vi "FipsAdjacent.vi"() -> (11 "Fips":i32[](array[numeric]))   [LabVIEW 2017] (continued)
 SD\"\t46127\t\"Sioux County, IA\"\t19167\n\"Union County, SD\"\t46127\t\"Woodbury County, IA\"\t19193\n\"Union County, SD\"\t46127\t\"Dakota County, NE\"\t31043\n\"Union County, SD\"\t46127\t\"Dixon County, NE\"\t31051\n\"Union County, SD\"\t46127\t\"Clay County, SD\"\t46027\n\"Union County, SD\"\t46127\t\"Lincoln County, SD\"\t46083\n\"Union County, SD\"\t46127\t\"Union County, SD\"\t46127\n\"Walworth County, SD\"\t46129\t\"Campbell County, SD\"\t46021\n\"Walworth County, SD\"\t46129\t\"Corson County, SD\"\t46031\n\"Walworth County, SD\"\t46129\t\"Dewey County, SD\"\t46041\n\"Walworth County, SD\"\t46129\t\"Edmunds County, SD\"\t46045\n\"Walworth County, SD\"\t46129\t\"McPherson County, SD\"\t46089\n\"Walworth County, SD\"\t46129\t\"Potter County, SD\"\t46107\n\"Walworth County, SD\"\t46129\t\"Walworth County, SD\"\t46129\n\"Yankton County, SD\"\t46135\t\"Cedar County, NE\"\t31027\n\"Yankton County, SD\"\t46135\t\"Knox County, NE\"\t31107\n\"Yankton County, SD\"\t46135\t\"Bon Homme County, SD\"\t46009\n\"Yankton County, SD\"\t46135\t\"Clay County, SD\"\t46027\n\"Yankton County, SD\"\t46135\t\"Hutchinson County, SD\"\t46067\n\"Yankton County, SD\"\t46135\t\"Turner County, SD\"\t46125\n\"Yankton County, SD\"\t46135\t\"Yankton County, SD\"\t46135\n\"Ziebach County, SD\"\t46137\t\"Corson County, SD\"\t46031\n\"Ziebach County, SD\"\t46137\t\"Dewey County, SD\"\t46041\n\"Ziebach County, SD\"\t46137\t\"Haakon County, SD\"\t46055\n\"Ziebach County, SD\"\t46137\t\"Meade County, SD\"\t46093\n\"Ziebach County, SD\"\t46137\t\"Perkins County, SD\"\t46105\n\"Ziebach County, SD\"\t46137\t\"Stanley County, SD\"\t46117\n\"Ziebach County, SD\"\t46137\t\"Ziebach County, SD\"\t46137\n\"Anderson County, TN\"\t47001\t\"Anderson County, TN\"\t47001\n\"Anderson County, TN\"\t47001\t\"Campbell County, TN\"\t47013\n\"Anderson County, TN\"\t47001\t\"Knox County, TN\"\t47093\n\"Anderson County, TN\"\t47001\t\"Morgan County, TN\"\t47129\n\"Anderson County, TN\"\t47001\t\"Roane County, TN\"\t47145\n\"Anderson County, TN\"\t47001\t\"Scott County, TN\"\t47151\n\"Anderson County, TN\"\t47001\t\"Union County, TN\"\t47173\n\"Bedford County, TN\"\t47003\t\"Bedford County, TN\"\t47003\n\"Bedford County, TN\"\t47003\t\"Coffee County, TN\"\t47031\n\"Bedford County, TN\"\t47003\t\"Lincoln County, TN\"\t47103\n\"Bedford County, TN\"\t47003\t\"Marshall County, TN\"\t47117\n\"Bedford County, TN\"\t47003\t\"Moore County, TN\"\t47127\n\"Bedford County, TN\"\t47003\t\"Rutherford County, TN\"\t47149\n\"Benton County, TN\"\t47005\t\"Benton County, TN\"\t47005\n\"Benton County, TN\"\t47005\t\"Carroll County, TN\"\t47017\n\"Benton County, TN\"\t47005\t\"Decatur County, TN\"\t47039\n\"Benton County, TN\"\t47005\t\"Henry County, TN\"\t47079\n\"Benton County, TN\"\t47005\t\"Houston County, TN\"\t47083\n\"Benton County, TN\"\t47005\t\"Humphreys County, TN\"\t47085\n\"Benton County, TN\"\t47005\t\"Perry County, TN\"\t47135\n\"Benton County, TN\"\t47005\t\"Stewart County, TN\"\t47161\n\"Bledsoe County, TN\"\t47007\t\"Bledsoe County, TN\"\t47007\n\"Bledsoe County, TN\"\t47007\t\"Cumberland County, TN\"\t47035\n\"Bledsoe County, TN\"\t47007\t\"Hamilton County, TN\"\t47065\n\"Bledsoe County, TN\"\t47007\t\"Rhea County, TN\"\t47143\n\"Bledsoe County, TN\"\t47007\t\"Sequatchie County, TN\"\t47153\n\"Bledsoe County, TN\"\t47007\t\"Van Buren County, TN\"\t47175\n\"Blount County, TN\"\t47009\t\"Graham County, NC\"\t37075\n\"Blount County, TN\"\t47009\t\"Swain County, NC\"\t37173\n\"Blount County, TN\"\t47009\t\"Blount County, TN\"\t47009\n\"Blount County, TN\"\t47009\t\"Knox County, TN\"\t47093\n\"Blount County, TN\"\t47009\t\"Loudon County, TN\"\t47105\n\"Blount County, TN\"\t47009\t\"Monroe County, TN\"\t47123\n\"Blount County, TN\"\t47009\t\"Sevier County, TN\"\t47155\n\"Bradley County, TN\"\t47011\t\"Murray County, GA\"\t13213\n\"Bradley County, TN\"\t47011\t\"Whitfield County, GA\"\t13313\n\"Bradley County, TN\"\t47011\t\"Bradley County, TN\"\t47011\n\"Bradley County, TN\"\t47011\t\"Hamilton County, TN\"\t47065\n\"Bradley County, TN\"\t47011\t\"McMinn County, TN\"\t47107\n\"Bradley County, TN\"\t47011\t\"Meigs County, TN\"\t47121\n\"Bradley County, TN\"\t47011\t\"Polk County, TN\"\t47139\n\"Campbell County, TN\"\t47013\t\"McCreary County, KY\"\t21147\n\"Campbell County, TN\"\t47013\t\"Whitley County, KY\"\t21235\n\"Campbell County, TN\"\t47013\t\"Anderson County, TN\"\t47001\n\"Campbell County, TN\"\t47013\t\"Campbell County, TN\"\t47013\n\"Campbell County, TN\"\t47013\t\"Claiborne County, TN\"\t47025\n\"Campbell County, TN\"\t47013\t\"Scott County, TN\"\t47151\n\"Campbell County, TN\"\t47013\t\"Union County, TN\"\t47173\n\"Cannon County, TN\"\t47015\t\"Cannon County, TN\"\t47015\n\"Cannon County, TN\"\t47015\t\"Coffee County, TN\"\t47031\n\"Cannon County, TN\"\t47015\t\"DeKalb County, TN\"\t47041\n\"Cannon County, TN\"\t47015\t\"Rutherford County, TN\"\t47149\n\"Cannon County, TN\"\t47015\t\"Warren County, TN\"\t47177\n\"Cannon County, TN\"\t47015\t\"Wilson County, TN\"\t47189\n\"Carroll County, TN\"\t47017\t\"Benton County, TN\"\t47005\n\"Carroll County, TN\"\t47017\t\"Carroll County, TN\"\t47017\n\"Carroll County, TN\"\t47017\t\"Decatur County, TN\"\t47039\n\"Carroll County, TN\"\t47017\t\"Gibson County, TN\"\t47053\n\"Carroll County, TN\"\t47017\t\"Henderson County, TN\"\t47077\n\"Carroll County, TN\"\t47017\t\"Henry County, TN\"\t47079\n\"Carroll County, TN\"\t47017\t\"Madison County, TN\"\t47113\n\"Carroll County, TN\"\t47017\t\"Weakley County, TN\"\t47183\n\"Carter County, TN\"\t47019\t\"Avery County, NC\"\t37011\n\"Carter County, TN\"\t47019\t\"Mitchell County, NC\"\t37121\n\"Carter County, TN\"\t47019\t\"Carter County, TN\"\t47019\n\"Carter County, TN\"\t47019\t\"Johnson County, TN\"\t47091\n\"Carter County, TN\"\t47019\t\"Sullivan County, TN\"\t47163\n\"Carter County, TN\"\t47019\t\"Unicoi County, TN\"\t47171\n\"Carter County, TN\"\t47019\t\"Washington County, TN\"\t47179\n\"Cheatham County, TN\"\t47021\t\"Cheatham County, TN\"\t47021\n\"Cheatham County, TN\"\t47021\t\"Davidson County, TN\"\t47037\n\"Cheatham County, TN\"\t47021\t\"Dickson County, TN\"\t47043\n\"Cheatham County, TN\"\t47021\t\"Montgomery County, TN\"\t47125\n\"Cheatham County, TN\"\t47021\t\"Robertson County, TN\"\t47147\n\"Cheatham County, TN\"\t47021\t\"Williamson County, TN\"\t47187\n\"Chester County, TN\"\t47023\t\"Chester County, TN\"\t47023\n\"Chester County, TN\"\t47023\t\"Hardeman County, TN\"\t47069\n\"Chester County, TN\"\t47023\t\"Hardin County, TN\"\t47071\n\"Chester County, TN\"\t47023\t\"Henderson County, TN\"\t47077\n\"Chester County, TN\"\t47023\t\"McNairy County, TN\"\t47109\n\"Chester County, TN\"\t47023\t\"Madison County, TN\"\t47113\n\"Claiborne County, TN\"\t47025\t\"Bell County, KY\"\t21013\n\"Claiborne County, TN\"\t47025\t\"Whitley County, KY\"\t21235\n\"Claiborne County, TN\"\t47025\t\"Campbell County, TN\"\t47013\n\"Claiborne County, TN\"\t47025\t\"Claiborne County, TN\"\t47025\n\"Claiborne County, TN\"\t47025\t\"Grainger County, TN\"\t47057\n\"Claiborne County, TN\"\t47025\t\"Hancock County, TN\"\t47067\n\"Claiborne County, TN\"\t47025\t\"Union County, TN\"\t47173\n\"Claiborne County, TN\"\t47025\t\"Lee County, VA\"\t51105\n\"Clay County, TN\"\t47027\t\"Clinton County, KY\"\t21053\n\"Clay County, TN\"\t47027\t\"Cumberland County, KY\"\t21057\n\"Clay County, TN\"\t47027\t\"Monroe County, KY\"\t21171\n\"Clay County, TN\"\t47027\t\"Clay County, TN\"\t47027\n\"Clay County, TN\"\t47027\t\"Jackson County, TN\"\t47087\n\"Clay County, TN\"\t47027\t\"Macon County, TN\"\t47111\n\"Clay County, TN\"\t47027\t\"Overton County, TN\"\t47133\n\"Clay County, TN\"\t47027\t\"Pickett County, TN\"\t47137\n\"Cocke County, TN\"\t47029\t\"Haywood County, NC\"\t37087\n\"Cocke County, TN\"\t47029\t\"Madison County, NC\"\t37115\n\"Cocke County, TN\"\t47029\t\"Cocke County, TN\"\t47029\n\"Cocke County, TN\"\t47029\t\"Greene County, TN\"\t47059\n\"Cocke County, TN\"\t47029\t\"Hamblen County, TN\"\t47063\n\"Cocke County, TN\"\t47029\t\"Jefferson County, TN\"\t47089\n\"Cocke County, TN\"\t47029\t\"Sevier County, TN\"\t47155\n\"Coffee County, TN\"\t47031\t\"Bedford County, TN\"\t47003\n\"Coffee County, TN\"\t47031\t\"Cannon County, TN\"\t47015\n\"Coffee County, TN\"\t47031\t\"Coffee County, TN\"\t47031\n\"Coffee County, TN\"\t47031\t\"Franklin County, TN\"\t47051\n\"Coffee County, TN\"\t47031\t\"Grundy County, TN\"\t47061\n\"Coffee County, TN\"\t47031\t\"Moore County, TN\"\t47127\n\"Coffee County, TN\"\t47031\t\"Rutherford County, TN\"\t47149\n\"Coffee County, TN\"\t47031\t\"Warren County, TN\"\t47177\n\"Crockett County, TN\"\t47033\t\"Crockett County, TN\"\t47033\n\"Crockett County, TN\"\t47033\t\"Dyer County, TN\"\t47045\n\"Crockett County, TN\"\t47033\t\"Gibson County, TN\"\t47053\n\"Crockett County, TN\"\t47033\t\"Haywood County, TN\"\t47075\n\"Crockett County, TN\"\t47033\t\"Lauderdale County, TN\"\t47097\n\"Crockett County, TN\"\t47033\t\"Madison County, TN\"\t47113\n\"Cumberland County, TN\"\t47035\t\"Bledsoe County, TN\"\t47007\n\"Cumberland County, TN\"\t47035\t\"Cumberland County, TN\"\t47035\n\"Cumberland County, TN\"\t47035\t\"Fentress County, TN\"\t47049\n\"Cumberland County, TN\"\t47035\t\"Morgan County, TN\"\t47129\n\"Cumberland County, TN\"\t47035\t\"Putnam County, TN\"\t47141\n\"Cumberland County, TN\"\t47035\t\"Rhea County, TN\"\t47143\n\"Cumberland County, TN\"\t47035\t\"Roane County, TN\"\t47145\n\"Cumberland County, TN\"\t47035\t\"Van Buren County, TN\"\t47175\n\"Cumberland County, TN\"\t47035\t\"White County, TN\"\t47185\n\"Davidson County, TN\"\t47037\t\"Cheatham County, TN\"\t47021\n\"Davidson County, TN\"\t47037\t\"Davidson County, TN\"\t47037\n\"Davidson County, TN\"\t47037\t\"Robertson County, TN\"\t47147\n\"Davidson County, TN\"\t47037\t\"Rutherford County, TN\"\t47149\n\"Davidson County, TN\"\t47037\t\"Sumner County, TN\"\t47165\n\"Davidson County, TN\"\t47037\t\"Williamson County, TN\"\t47187\n\"Davidson County, TN\"\t47037\t\"Wilson County, TN\"\t47189\n\"Decatur County, TN\"\t47039\t\"Benton County, TN\"\t47005\n\"Decatur County, TN\"\t47039\t\"Carroll County, TN\"\t47017\n\"Decatur County, TN\"\t47039\t\"Decatur County, TN\"\t47039\n\"Decatur County, TN\"\t47039\t\"Hardin County, TN\"\t47071\n\"Decatur County, TN\"\t47039\t\"Henderson County, TN\"\t47077\n\"Decatur County, TN\"\t47039\t\"Perry County, TN\"\t47135\n\"Decatur County, TN\"\t47039\t\"Wayne County, TN\"\t47181\n\"DeKalb County, TN\"\t47041\t\"Cannon County, TN\"\t47015\n\"DeKalb County, TN\"\t47041\t\"DeKalb County, TN\"\t47041\n\"DeKalb County, TN\"\t47041\t\"Putnam County, TN\"\t47141\n\"DeKalb County, TN\"\t47041\t\"Smith County, TN\"\t47159\n\"DeKalb County, TN\"\t47041\t\"Warren County, TN\"\t47177\n\"DeKalb County, TN\"\t47041\t\"White County, TN\"\t47185\n\"DeKalb County, TN\"\t47041\t\"Wilson County, TN\"\t47189\n\"Dickson County, TN\"\t47043\t\"Cheatham County, TN\"\t47021\n\"Dickson County, TN\"\t47043\t\"Dickson County, TN\"\t47043\n\"Dickson County, TN\"\t47043\t\"Hickman County, TN\"\t47081\n\"Dickson County, TN\"\t47043\t\"Houston County, TN\"\t47083\n\"Dickson County, TN\"\t47043\t\"Humphreys County, TN\"\t47085\n\"Dickson County, TN\"\t47043\t\"Montgomery County, TN\"\t47125\n\"Dickson County, TN\"\t47043\t\"Williamson County, TN\"\t47187\n\"Dyer County, TN\"\t47045\t\"Mississippi County, AR\"\t05093\n\"Dyer County, TN\"\t47045\t\"Pemiscot County, MO\"\t29155\n\"Dyer County, TN\"\t47045\t\"Crockett County, TN\"\t47033\n\"Dyer County, TN\"\t47045\t\"Dyer County, TN\"\t47045\n\"Dyer County, TN\"\t47045\t\"Gibson County, TN\"\t47053\n\"Dyer County, TN\"\t47045\t\"Lake County, TN\"\t47095\n\"Dyer County, TN\"\t47045\t\"Lauderdale County, TN\"\t47097\n\"Dyer County, TN\"\t47045\t\"Obion County, TN\"\t47131\n\"Fayette County, TN\"\t47047\t\"Benton County, MS\"\t28009\n\"Fayette County, TN\"\t47047\t\"Marshall County, MS\"\t28093\n\"Fayette County, TN\"\t47047\t\"Fayette County, TN\"\t47047\n\"Fayette County, TN\"\t47047\t\"Hardeman County, TN\"\t47069\n\"Fayette County, TN\"\t47047\t\"Haywood County, TN\"\t47075\n\"Fayette County, TN\"\t47047\t\"Shelby County, TN\"\t47157\n\"Fayette County, TN\"\t47047\t\"Tipton County, TN\"\t47167\n\"Fentress County, TN\"\t47049\t\"Cumberland County, TN\"\t47035\n\"Fentress County, TN\"\t47049\t\"Fentress County, TN\"\t47049\n\"Fentress County, TN\"\t47049\t\"Morgan County, TN\"\t47129\n\"Fentress County, TN\"\t47049\t\"Overton County, TN\"\t47133\n\"Fentress County, TN\"\t47049\t\"Pickett County, TN\"\t47137\n\"Fentress County, TN\"\t47049\t\"Putnam County, TN\"\t47141\n\"Fentress County, TN\"\t47049\t\"Scott County, TN\"\t47151\n\"Franklin County, TN\"\t47051\t\"Jackson County, AL\"\t01071\n\"Franklin County, TN\"\t47051\t\"Madison County, AL\"\t01089\n\"Franklin County, TN\"\t47051\t\"Coffee County, TN\"\t47031\n\"Franklin County, TN\"\t47051\t\"Franklin County, TN\"\t47051\n\"Franklin County, TN\"\t47051\t\"Grundy County, TN\"\t47061\n\"Franklin County, TN\"\t47051\t\"Lincoln County, TN\"\t47103\n\"Franklin County, TN\"\t47051\t\"Marion County, TN\"\t47115\n\"Franklin County, TN\"\t47051\t\"Moore County, TN\"\t47127\n\"Gibson County, TN\"\t47053\t\"Carroll County, TN\"\t47017\n\"Gibson County, TN\"\t47053\t\"Crockett County, TN\"\t47033\n\"Gibson County, TN\"\t47053\t\"Dyer County, TN\"\t47045\n\"Gibson County, TN\"\t47053\t\"Gibson County, TN\"\t47053\n\"Gibson County, TN\"\t47053\t\"Madison County, TN\"\t47113\n\"Gibson County, TN\"\t47053\t\"Obion County, TN\"\t47131\n\"Gibson County, TN\"\t47053\t\"Weakley County, TN\"\t47183\n\"Giles County, TN\"\t47055\t\"Lauderdale County, AL\"\t01077\n\"Giles County, TN\"\t47055\t\"Limestone County, AL\"\t01083\n\"Giles County, TN\"\t47055\t\"Giles County, TN\"\t47055\n\"Giles County, TN\"\t47055\t\"Lawrence County, TN\"\t47099\n\"Giles County, TN\"\t47055\t\"Lincoln County, TN\"\t47103\n\"Giles County, TN\"\t47055\t\"Marshall County, TN\"\t47117\n\"Giles County, TN\"\t47055\t\"Maury County, TN\"\t47119\n\"Grainger County, TN\"\t47057\t\"Claiborne County, TN\"\t47025\n\"Grainger County, TN\"\t47057\t\"Grainger County, TN\"\t47057\n\"Grainger County, TN\"\t47057\t\"Hamblen County, TN\"\t47063\n\"Grainger County, TN\"\t47057\t\"Hancock County, TN\"\t47067\n\"Grainger County, TN\"\t47057\t\"Hawkins County, TN\"\t47073\n\"Grainger County, TN\"\t47057\t\"Jefferson County, TN\"\t47089\n\"Grainger County, TN\"\t47057\t\"Knox County, TN\"\t47093\n\"Grainger County, TN\"\t47057\t\"Union County, TN\"\t47173\n\"Greene County, TN\"\t47059\t\"Madison County, NC\"\t37115\n\"Greene County, TN\"\t47059\t\"Cocke County, TN\"\t47029\n\"Greene County, TN\"\t47059\t\"Greene County, TN\"\t47059\n\"Greene County, TN\"\t47059\t\"Hamblen County, TN\"\t47063\n\"Greene County, TN\"\t47059\t\"Hawkins County, TN\"\t47073\n\"Greene County, TN\"\t47059\t\"Unicoi County, TN\"\t47171\n\"Greene County, TN\"\t47059\t\"Washington County, TN\"\t47179\n\"Grundy County, TN\"\t47061\t\"Coffee County, TN\"\t47031\n\"Grundy County, TN\"\t47061\t\"Franklin County, TN\"\t47051\n\"Grundy County, TN\"\t47061\t\"Grundy County, TN\"\t47061\n\"Grundy County, TN\"\t47061\t\"Marion County, TN\"\t47115\n\"Grundy County, TN\"\t47061\t\"Sequatchie County, TN\"\t47153\n\"Grundy County, TN\"\t47061\t\"Warren County, TN\"\t47177\n\"Hamblen County, TN\"\t47063\t\"Cocke County, TN\"\t47029\n\"Hamblen County, TN\"\t47063\t\"Grainger County, TN\"\t47057\n\"Hamblen County, TN\"\t47063\t\"Greene County, TN\"\t47059\n\"Hamblen County, TN\"\t47063\t\"Hamblen County, TN\"\t47063\n\"Hamblen County, TN\"\t47063\t\"Hawkins County, TN\"\t47073\n\"Hamblen County, TN\"\t47063\t\"Jefferson County, TN\"\t47089\n\"Hamilton County, TN\"\t47065\t\"Catoosa County, GA\"\t13047\n\"Hamilton County, TN\"\t47065\t\"Dade County, GA\"\t13083\n\"Hamilton County, TN\"\t47065\t\"Walker County, GA\"\t13295\n\"Hamilton County, TN\"\t47065\t\"Whitfield County, GA\"\t13313\n\"Hamilton County, TN\"\t47065\t\"Bledsoe County, TN\"\t47007\n\"Hamilton County, TN\"\t47065\t\"Bradley County, TN\"\t47011\n\"Hamilton County, TN\"\t47065\t\"Hamilton County, TN\"\t47065\n\"Hamilton County, TN\"\t47065\t\"Marion County, TN\"\t47115\n\"Hamilton County, TN\"\t47065\t\"Meigs County, TN\"\t47121\n\"Hamilton County, TN\"\t47065\t\"Rhea County, TN\"\t47143\n\"Hamilton County, TN\"\t47065\t\"Sequatchie County, TN\"\t47153\n\"Hancock County, TN\"\t47067\t\"Claiborne County, TN\"\t47025\n\"Hancock County, TN\"\t47067\t\"Grainger County, TN\"\t47057\n\"Hancock County, TN\"\t47067\t\"Hancock County, TN\"\t47067\n\"Hancock County, TN\"\t47067\t\"Hawkins County, TN\"\t47073\n\"Hancock County, TN\"\t47067\t\"Lee County, VA\"\t51105\n\"Hancock County, TN\"\t47067\t\"Scott County, VA\"\t51169\n\"Hardeman County, TN\"\t47069\t\"Alcorn County, MS\"\t28003\n\"Hardeman County, TN\"\t47069\t\"Benton County, MS\"\t28009\n\"Hardeman County, TN\"\t47069\t\"Tippah County, MS\"\t28139\n\"Hardeman County, TN\"\t47069\t\"Chester County, TN\"\t47023\n\"Hardeman County, TN\"\t47069\t\"Fayette County, TN\"\t47047\n\"Hardeman County, TN\"\t47069\t\"Hardeman County, TN\"\t47069\n\"Hardeman County, TN\"\t47069\t\"Haywood County, TN\"\t47075\n\"Hardeman County, TN\"\t47069\t\"McNairy County, TN\"\t47109\n\"Hardeman County, TN\"\t47069\t\"Madison County, TN\"\t47113\n\"Hardin County, TN\"\t47071\t\"Lauderdale County, AL\"\t01077\n\"Hardin County, TN\"\t47071\t\"Alcorn County, MS\"\t28003\n\"Hardin County, TN\"\t47071\t\"Tishomingo County, MS\"\t28141\n\"Hardin County, TN\"\t47071\t\"Chester County, TN\"\t47023\n\"Hardin County, TN\"\t47071\t\"Decatur County, TN\"\t47039\n\"Hardin County, TN\"\t47071\t\"Hardin County, TN\"\t47071\n\"Hardin County, TN\"\t47071\t\"Henderson County, TN\"\t47077\n\"Hardin County, TN\"\t47071\t\"McNairy County, TN\"\t47109\n\"Hardin County, TN\"\t47071\t\"Wayne County, TN\"\t47181\n\"Hawkins County, TN\"\t47073\t\"Grainger County, TN\"\t47057\n\"Hawkins County, TN\"\t47073\t\"Greene County, TN\"\t47059\n\"Hawkins County, TN\"\t47073\t\"Hamblen County, TN\"\t47063\n\"Hawkins County, TN\"\t47073\t\"Hancock County, TN\"\t47067\n\"Hawkins County, TN\"\t47073\t\"Hawkins County, TN\"\t47073\n\"Hawkins County, TN\"\t47073\t\"Sullivan County, TN\"\t47163\n\"Hawkins County, TN\"\t47073\t\"Washington County, TN\"\t47179\n\"Hawkins County, TN\"\t47073\t\"Scott County, VA\"\t51169\n\"Haywood County, TN\"\t47075\t\"Crockett County, TN\"\t47033\n\"Haywood County, TN\"\t47075\t\"Fayette County, TN\"\t47047\n\"Haywood County, TN\"\t47075\t\"Hardeman County, TN\"\t47069\n\"Haywood County, TN\"\t47075\t\"Haywood County, TN\"\t47075\n\"Haywood County, TN\"\t47075\t\"Lauderdale County, TN\"\t47097\n\"Haywood County, TN\"\t47075\t\"Madison County, TN\"\t47113\n\"Haywood County, TN\"\t47075\t\"Tipton County, TN\"\t47167\n\"Henderson County, TN\"\t47077\t\"Carroll County, TN\"\t47017\n\"Henderson County, TN\"\t47077\t\"Chester County, TN\"\t47023\n\"Henderson County, TN\"\t47077\t\"Decatur County, TN\"\t47039\n\"Henderson County, TN\"\t47077\t\"Hardin County, TN\"\t47071\n\"Henderson County, TN\"\t47077\t\"Henderson County, TN\"\t47077\n\"Henderson County, TN\"\t47077\t\"Madison County, TN\"\t47113\n\"Henry County, TN\"\t47079\t\"Calloway County, KY\"\t21035\n\"Henry County, TN\"\t47079\t\"Graves County, KY\"\t21083\n\"Henry County, TN\"\t47079\t\"Benton County, TN\"\t47005\n\"Henry County, TN\"\t47079\t\"Carroll County, TN\"\t47017\n\"Henry County, TN\"\t47079\t\"Henry County, TN\"\t47079\n\"Henry County, TN\"\t47079\t\"Stewart County, TN\"\t47161\n\"Henry County, TN\"\t47079\t\"Weakley County, TN\"\t47183\n\"Hickman County, TN\"\t47081\t\"Dickson County, TN\"\t47043\n\"Hickman County, TN\"\t47081\t\"Hickman County, TN\"\t47081\n\"Hickman County, TN\"\t47081\t\"Humphreys County, TN\"\t47085\n\"Hickman County, TN\"\t47081\t\"Lewis County, TN\"\t47101\n\"Hickman County, TN\"\t47081\t\"Maury County, TN\"\t47119\n\"Hickman County, TN\"\t47081\t\"Perry County, TN\"\t47135\n\"Hickman County, TN\"\t47081\t\"Williamson County, TN\"\t47187\n\"Houston County, TN\"\t47083\t\"Benton County, TN\"\t47005\n\"Houston County, TN\"\t47083\t\"Dickson County, TN\"\t47043\n\"Houston County, TN\"\t47083\t\"Houston County, TN\"\t47083\n\"Houston County, TN\"\t47083\t\"Humphreys County, TN\"\t47085\n\"Houston County, TN\"\t47083\t\"Montgomery County, TN\"\t47125\n\"Houston County, TN\"\t47083\t\"Stewart County, TN\"\t47161\n\"Humphreys County, TN\"\t47085\t\"Benton County, TN\"\t47005\n\"Humphreys County, TN\"\t47085\t\"Dickson County, TN\"\t47043\n\"Humphreys County, TN\"\t47085\t\"Hickman County, TN\"\t47081\n\"Humphreys County, TN\"\t47085\t\"Houston County, TN\"\t47083\n\"Humphreys County, TN\"\t47085\t\"Humphreys County, TN\"\t47085\n\"Humphreys County, TN\"\t47085\t\"Perry County, TN\"\t47135\n\"Jackson County, TN\"\t47087\t\"Clay County, TN\"\t47027\n\"Jackson County, TN\"\t47087\t\"Jackson County, TN\"\t47087\n\"Jackson County, TN\"\t47087\t\"Macon County, TN\"\t47111\n\"Jackson County, TN\"\t47087\t\"Overton County, TN\"\t47133\n\"Jackson County, TN\"\t47087\t\"Putnam County, TN\"\t47141\n\"Jackson County, TN\"\t47087\t\"Smith County, TN\"\t47159\n\"Jefferson County, TN\"\t47089\t\"Cocke County, TN\"\t47029\n\"Jefferson County, TN\"\t47089\t\"Grainger County, TN\"\t47057\n\"Jefferson County, TN\"\t47089\t\"Hamblen County, TN\"\t47063\n\"Jefferson County, TN\"\t47089\t\"Jefferson County, TN\"\t47089\n\"Jefferson County, TN\"\t47089\t\"Knox County, TN\"\t47093\n\"Jefferson County, TN\"\t47089\t\"Sevier County, TN\"\t47155\n\"Johnson County, TN\"\t47091\t\"Ashe County, NC\"\t37009\n\"Johnson County, TN\"\t47091\t\"Avery County, NC\"\t37011\n\"Johnson County, TN\"\t47091\t\"Watauga County, NC\"\t37189\n\"Johnson County, TN\"\t47091\t\"Carter County, TN\"\t47019\n\"Johnson County, TN\"\t47091\t\"Johnson County, TN\"\t47091\n\"Johnson County, TN\"\t47091\t\"Sullivan County, TN\"\t47163\n\"Johnson County, TN\"\t47091\t\"Grayson County, VA\"\t51077\n\"Johnson County, TN\"\t47091\t\"Washington County, VA\"\t51191\n\"Knox County, TN\"\t47093\t\"Anderson County, TN\"\t47001\n\"Knox County, TN\"\t47093\t\"Blount County, TN\"\t47009\n\"Knox County, TN\"\t47093\t\"Grainger County, TN\"\t47057\n\"Knox County, TN\"\t47093\t\"Jefferson County, TN\"\t47089\n\"Knox County, TN\"\t47093\t\"Knox County, TN\"\t47093\n\"Knox County, TN\"\t47093\t\"Loudon County, TN\"\t47105\n\"Knox County, TN\"\t47093\t\"Roane County, TN\"\t47145\n\"Knox County, TN\"\t47093\t\"Sevier County, TN\"\t47155\n\"Knox County, TN\"\t47093\t\"Union County, TN\"\t47173\n\"Lake County, TN\"\t47095\t\"Fulton County, KY\"\t21075\n\"Lake County, TN\"\t47095\t\"New Madrid County, MO\"\t29143\n\"Lake County, TN\"\t47095\t\"Pemiscot County, MO\"\t29155\n\"Lake County, TN\"\t47095\t\"Dyer County, TN\"\t47045\n\"Lake County, TN\"\t47095\t\"Lake County, TN\"\t47095\n\"Lake County, TN\"\t47095\t\"Obion County, TN\"\t47131\n\"Lauderdale County, TN\"\t47097\t\"Mississippi County, AR\"\t05093\n\"Lauderdale County, TN\"\t47097\t\"Crockett County, TN\"\t47033\n\"Lauderdale County, TN\"\t47097\t\"Dyer County, TN\"\t47045\n\"Lauderdale County, TN\"\t47097\t\"Haywood County, TN\"\t47075\n\"Lauderdale County, TN\"\t47097\t\"Lauderdale County, TN\"\t47097\n\"Lauderdale County, TN\"\t47097\t\"Tipton County, TN\"\t47167\n\"Lawrence County, TN\"\t47099\t\"Lauderdale County, AL\"\t01077\n\"Lawrence County, TN\"\t47099\t\"Giles County, TN\"\t47055\n\"Lawrence County, TN\"\t47099\t\"Lawrence County, TN\"\t47099\n\"Lawrence County, TN\"\t47099\t\"Lewis County, TN\"\t47101\n\"Lawrence County, TN\"\t47099\t\"Maury County, TN\"\t47119\n\"Lawrence County, TN\"\t47099\t\"Wayne County, TN\"\t47181\n\"Lewis County, TN\"\t47101\t\"Hickman County, TN\"\t47081\n\"Lewis County, TN\"\t47101\t\"Lawrence County, TN\"\t47099\n\"Lewis County, TN\"\t47101\t\"Lewis County, TN\"\t47101\n\"Lewis County, TN\"\t47101\t\"Maury County, TN\"\t47119\n\"Lewis County, TN\"\t47101\t\"Perry County, TN\"\t47135\n\"Lewis County, TN\"\t47101\t\"Wayne County, TN\"\t47181\n\"Lincoln County, TN\"\t47103\t\"Limestone County, AL\"\t01083\n\"Lincoln County, TN\"\t47103\t\"Madison County, AL\"\t01089\n\"Lincoln County, TN\"\t47103\t\"Bedford County, TN\"\t47003\n\"Lincoln County, TN\"\t47103\t\"Franklin County, TN\"\t47051\n\"Lincoln County, TN\"\t47103\t\"Giles County, TN\"\t47055\n\"Lincoln County, TN\"\t47103\t\"Lincoln County, TN\"\t47103\n\"Lincoln County, TN\"\t47103\t\"Marshall County, TN\"\t47117\n\"Lincoln County, TN\"\t47103\t\"Moore County, TN\"\t47127\n\"Loudon County, TN\"\t47105\t\"Blount County, TN\"\t47009\n\"Loudon County, TN\"\t47105\t\"Knox County, TN\"\t47093\n\"Loudon County, TN\"\t47105\t\"Loudon County, TN\"\t47105\n\"Loudon County, TN\"\t47105\t\"McMinn County, TN\"\t47107\n\"Loudon County, TN\"\t47105\t\"Monroe County, TN\"\t47123\n\"Loudon County, TN\"\t47105\t\"Roane County, TN\"\t47145\n\"McMinn County, TN\"\t47107\t\"Bradley County, TN\"\t47011\n\"McMinn County, TN\"\t47107\t\"Loudon County, TN\"\t47105\n\"McMinn County, TN\"\t47107\t\"McMinn County, TN\"\t47107\n\"McMinn County, TN\"\t47107\t\"Meigs County, TN\"\t47121\n\"McMinn County, TN\"\t47107\t\"Monroe County, TN\"\t47123\n\"McMinn County, TN\"\t47107\t\"Polk County, TN\"\t47139\n\"McMinn County, TN\"\t47107\t\"Roane County, TN\"\t47145\n\"McNairy County, TN\"\t47109\t\"Alcorn County, MS\"\t28003\n\"McNairy County, TN\"\t47109\t\"Chester County, TN\"\t47023\n\"McNairy County, TN\"\t47109\t\"Hardeman County, TN\"\t47069\n\"McNairy County, TN\"\t47109\t\"Hardin County, TN\"\t47071\n\"McNairy County, TN\"\t47109\t\"McNairy County, TN\"\t47109\n\"Macon County, TN\"\t47111\t\"Allen County, KY\"\t21003\n\"Macon County, TN\"\t47111\t\"Monroe County, KY\"\t21171\n\"Macon County, TN\"\t47111\t\"Clay County, TN\"\t47027\n\"Macon County, TN\"\t47111\t\"Jackson County, TN\"\t47087\n\"Macon County, TN\"\t47111\t\"Macon County, TN\"\t47111\n\"Macon County, TN\"\t47111\t\"Smith County, TN\"\t47159\n\"Macon County, TN\"\t47111\t\"Sumner County, TN\"\t47165\n\"Macon County, TN\"\t47111\t\"Trousdale County, TN\"\t47169\n\"Madison County, TN\"\t47113\t\"Carroll County, TN\"\t47017\n\"Madison County, TN\"\t47113\t\"Chester County, TN\"\t47023\n\"Madison County, TN\"\t47113\t\"Crockett County, TN\"\t47033\n\"Madison County, TN\"\t47113\t\"Gibson County, TN\"\t47053\n\"Madison County, TN\"\t47113\t\"Hardeman County, TN\"\t47069\n\"Madison County, TN\"\t47113\t\"Haywood County, TN\"\t47075\n\"Madison County, TN\"\t47113\t\"Henderson County, TN\"\t47077\n\"Madison County, TN\"\t47113\t\"Madison County, TN\"\t47113\n\"Marion County, TN\"\t47115\t\"Jackson County, AL\"\t01071\n\"Marion County, TN\"\t47115\t\"Dade County, GA\"\t13083\n\"Marion County, TN\"\t47115\t\"Franklin County, TN\"\t47051\n\"Marion County, TN\"\t47115\t\"Grundy County, TN\"\t47061\n\"Marion County, TN\"\t47115\t\"Hamilton County, TN\"\t47065\n\"Marion County, TN\"\t47115\t\"Marion County, TN\"\t47115\n\"Marion County, TN\"\t47115\t\"Sequatchie County, TN\"\t47153\n\"Marshall County, TN\"\t47117\t\"Bedford County, TN\"\t47003\n\"Marshall County, TN\"\t47117\t\"Giles County, TN\"\t47055\n\"Marshall County, TN\"\t47117\t\"Lincoln County, TN\"\t47103\n\"Marshall County, TN\"\t47117\t\"Marshall County, TN\"\t47117\n\"Marshall County, TN\"\t47117\t\"Maury County, TN\"\t47119\n\"Marshall County, TN\"\t47117\t\"Rutherford County, TN\"\t47149\n\"Marshall County, TN\"\t47117\t\"Williamson County, TN\"\t47187\n\"Maury County, TN\"\t47119\t\"Giles County, TN\"\t47055\n\"Maury County, TN\"\t47119\t\"Hickman County, TN\"\t47081\n\"Maury County, TN\"\t47119\t\"Lawrence County, TN\"\t47099\n\"Maury County, TN\"\t47119\t\"Lewis County, TN\"\t47101\n\"Maury County, TN\"\t47119\t\"Marshall County, TN\"\t47117\n\"Maury County, TN\"\t47119\t\"Maury County, TN\"\t47119\n\"Maury County, TN\"\t47119\t\"Williamson County, TN\"\t47187\n\"Meigs County, TN\"\t47121\t\"Bradley County, TN\"\t47011\n\"Meigs County, TN\"\t47121\t\"Hamilton County, TN\"\t47065\n\"Meigs County, TN\"\t47121\t\"McMinn County, TN\"\t47107\n\"Meigs County, TN\"\t47121\t\"Meigs County, TN\"\t47121\n\"Meigs County, TN\"\t47121\t\"Rhea County, TN\"\t47143\n\"Meigs County, TN\"\t47121\t\"Roane County, TN\"\t47145\n\"Monroe County, TN\"\t47123\t\"Cherokee County, NC\"\t37039\n\"Monroe County, TN\"\t47123\t\"Graham County, NC\"\t37075\n\"Monroe County, TN\"\t47123\t\"Blount County, TN\"\t47009\n\"Monroe County, TN\"\t47123\t\"Loudon County, TN\"\t47105\n\"Monroe County, TN\"\t47123\t\"McMinn County, TN\"\t47107\n\"Monroe County, TN\"\t47123\t\"Monroe County, TN\"\t47123\n\"Monroe County, TN\"\t47123\t\"Polk County, TN\"\t47139\n\"Montgomery County, TN\"\t47125\t\"Christian County, KY\"\t21047\n\"Montgomery County, TN\"\t47125\t\"Todd County, KY\"\t21219\n\"Montgomery County, TN\"\t47125\t\"Cheatham County, TN\"\t47021\n\"Montgomery County, TN\"\t47125\t\"Dickson County, TN\"\t47043\n\"Montgomery County, TN\"\t47125\t\"Houston County, TN\"\t47083\n\"Montgomery County, TN\"\t47125\t\"Montgomery County, TN\"\t47125\n\"Montgomery County, TN\"\t47125\t\"Robertson County, TN\"\t47147\n\"Montgomery County, TN\"\t47125\t\"Stewart County, TN\"\t47161\n\"Moore County, TN\"\t47127\t\"Bedford County, TN\"\t47003\n\"Moore County, TN\"\t47127\t\"Coffee County, TN\"\t47031\n\"Moore County, TN\"\t47127\t\"Franklin County, TN\"\t47051\n\"Moore County, TN\"\t47127\t\"Lincoln County, TN\"\t47103\n\"Moore County, TN\"\t47127\t\"Moore County, TN\"\t47127\n\"Morgan County, TN\"\t47129\t\"Anderson County, TN\"\t47001\n\"Morgan County, TN\"\t47129\t\"Cumberland County, TN\"\t47035\n\"Morgan County, TN\"\t47129\t\"Fentress County, TN\"\t47049\n\"Morgan County, TN\"\t47129\t\"Morgan County, TN\"\t47129\n\"Morgan County, TN\"\t47129\t\"Roane County, TN\"\t47145\n\"Morgan County, TN\"\t47129\t\"Scott County, TN\"\t47151\n\"Obion County, TN\"\t47131\t\"Fulton County, KY\"\t21075\n\"Obion County, TN\"\t47131\t\"Hickman County, KY\"\t21105\n\"Obion County, TN\"\t47131\t\"Dyer County, TN\"\t47045\n\"Obion County, TN\"\t47131\t\"Gibson County, TN\"\t47053\n\"Obion County, TN\"\t47131\t\"Lake County, TN\"\t47095\n\"Obion County, TN\"\t47131\t\"Obion County, TN\"\t47131\n\"Obion County, TN\"\t47131\t\"Weakley County, TN\"\t47183\n\"Overton County, TN\"\t47133\t\"Clay County, TN\"\t47027\n\"Overton County, TN\"\t47133\t\"Fentress County, TN\"\t47049\n\"Overton County, TN\"\t47133\t\"Jackson County, TN\"\t47087\n\"Overton County, TN\"\t47133\t\"Overton County, TN\"\t47133\n\"Overton County, TN\"\t47133\t\"Pickett County, TN\"\t47137\n\"Overton County, TN\"\t47133\t\"Putnam County, TN\"\t47141\n\"Perry County, TN\"\t47135\t\"Benton County, TN\"\t47005\n\"Perry County, TN\"\t47135\t\"Decatur County, TN\"\t47039\n\"Perry County, TN\"\t47135\t\"Hickman County, TN\"\t47081\n\"Perry County, TN\"\t47135\t\"Humphreys County, TN\"\t47085\n\"Perry County, TN\"\t47135\t\"Lewis County, TN\"\t47101\n\"Perry County, TN\"\t47135\t\"Perry County, TN\"\t47135\n\"Perry County, TN\"\t47135\t\"Wayne County, TN\"\t47181\n\"Pickett County, TN\"\t47137\t\"Clinton County, KY\"\t21053\n\"Pickett County, TN\"\t47137\t\"Wayne County, KY\"\t21231\n\"Pickett County, TN\"\t47137\t\"Clay County, TN\"\t47027\n\"Pickett County, TN\"\t47137\t\"Fentress County, TN\"\t47049\n\"Pickett County, TN\"\t47137\t\"Overton County, TN\"\t47133\n\"Pickett County, TN\"\t47137\t\"Pickett County, TN\"\t47137\n\"Pickett County, TN\"\t47137\t\"Scott County, TN\"\t47151\n\"Polk County, TN\"\t47139\t\"Fannin County, GA\"\t13111\n\"Polk County, TN\"\t47139\t\"Murray County, GA\"\t13213\n\"Polk County, TN\"\t47139\t\"Cherokee County, NC\"\t37039\n\"Polk County, TN\"\t47139\t\"Bradley County, TN\"\t47011\n\"Polk County, TN\"\t47139\t\"McMinn County, TN\"\t47107\n\"Polk County, TN\"\t47139\t\"Monroe County, TN\"\t47123\n\"Polk County, TN\"\t47139\t\"Polk County, TN\"\t47139\n\"Putnam County, TN\"\t47141\t\"Cumberland County, TN\"\t47035\n\"Putnam County, TN\"\t47141\t\"DeKalb County, TN\"\t47041\n\"Putnam County, TN\"\t47141\t\"Fentress County, TN\"\t47049\n\"Putnam County, TN\"\t47141\t\"Jackson County, TN\"\t47087\n\"Putnam County, TN\"\t47141\t\"Overton County, TN\"\t47133\n\"Putnam County, TN\"\t47141\t\"Putnam County, TN\"\t47141\n\"Putnam County, TN\"\t47141\t\"Smith County, TN\"\t47159\n\"Putnam County, TN\"\t47141\t\"White County, TN\"\t47185\n\"Rhea County, TN\"\t47143\t\"Bledsoe County, TN\"\t47007\n\"Rhea County, TN\"\t47143\t\"Cumberland County, TN\"\t47035\n\"Rhea County, TN\"\t47143\t\"Hamilton County, TN\"\t47065\n\"Rhea County, TN\"\t47143\t\"Meigs County, TN\"\t47121\n\"Rhea County, TN\"\t47143\t\"Rhea County, TN\"\t47143\n\"Rhea County, TN\"\t47143\t\"Roane County, TN\"\t47145\n\"Roane County, TN\"\t47145\t\"Anderson County, TN\"\t47001\n\"Roane County, TN\"\t47145\t\"Cumberland County, TN\"\t47035\n\"Roane County, TN\"\t47145\t\"Knox County, TN\"\t47093\n\"Roane County, TN\"\t47145\t\"Loudon County, TN\"\t47105\n\"Roane County, TN\"\t47145\t\"McMinn County, TN\"\t47107\n\"Roane County, TN\"\t47145\t\"Meigs County, TN\"\t47121\n\"Roane County, TN\"\t47145\t\"Morgan County, TN\"\t47129\n\"Roane County, TN\"\t47145\t\"Rhea County, TN\"\t47143\n\"Roane County, TN\"\t47145\t\"Roane County, TN\"\t47145\n\"Robertson County, TN\"\t47147\t\"Logan County, KY\"\t21141\n\"Robertson County, TN\"\t47147\t\"Simpson County, KY\"\t21213\n\"Robertson County, TN\"\t47147\t\"Todd County, KY\"\t21219\n\"Robertson County, TN\"\t47147\t\"Cheatham County, TN\"\t47021\n\"Robertson County, TN\"\t47147\t\"Davidson County, TN\"\t47037\n\"Robertson County, TN\"\t47147\t\"Montgomery County, TN\"\t47125\n\"Robertson County, TN\"\t47147\t\"Robertson County, TN\"\t47147\n\"Robertson County, TN\"\t47147\t\"Sumner County, TN\"\t47165\n\"Rutherford County, TN\"\t47149\t\"Bedford County, TN\"\t47003\n\"Rutherford County, TN\"\t47149\t\"Cannon County, TN\"\t47015\n\"Rutherford County, TN\"\t47149\t\"Coffee County, TN\"\t47031\n\"Rutherford County, TN\"\t47149\t\"Davidson County, TN\"\t47037\n\"Rutherford County, TN\"\t47149\t\"Marshall County, TN\"\t47117\n\"Rutherford County, TN\"\t47149\t\"Rutherford County, TN\"\t47149\n\"Rutherford County, TN\"\t47149\t\"Williamson County, TN\"\t47187\n\"Rutherford County, TN\"\t47149\t\"Wilson County, TN\"\t47189\n\"Scott County, TN\"\t47151\t\"McCreary County, KY\"\t21147\n\"Scott County, TN\"\t47151\t\"Wayne County, KY\"\t21231\n\"Scott County, TN\"\t47151\t\"Anderson County, TN\"\t47001\n\"Scott County, TN\"\t47151\t\"Campbell County, TN\"\t47013\n\"Scott County, TN\"\t47151\t\"Fentress County, TN\"\t47049\n\"Scott County, TN\"\t47151\t\"Morgan County, TN\"\t47129\n\"Scott County, TN\"\t47151\t\"Pickett County, TN\"\t47137\n\"Scott County, TN\"\t47151\t\"Scott County, TN\"\t47151\n\"Sequatchie County, TN\"\t47153\t\"Bledsoe County, TN\"\t47007\n\"Sequatchie County, TN\"\t47153\t\"Grundy County, TN\"\t47061\n\"Sequatchie County, TN\"\t47153\t\"Hamilton County, TN\"\t47065\n\"Sequatchie County, TN\"\t47153\t\"Marion County, TN\"\t47115\n\"Sequatchie County, TN\"\t47153\t\"Sequatchie County, TN\"\t47153\n\"Sequatchie County, TN\"\t47153\t\"Van Buren County, TN\"\t47175\n\"Sequatchie County, TN\"\t47153\t\"Warren County, TN\"\t47177\n\"Sevier County, TN\"\t47155\t\"Haywood County, NC\"\t37087\n\"Sevier County, TN\"\t47155\t\"Swain County, NC\"\t37173\n\"Sevier County, TN\"\t47155\t\"Blount County, TN\"\t47009\n\"Sevier County, TN\"\t47155\t\"Cocke County, TN\"\t47029\n\"Sevier County, TN\"\t47155\t\"Jefferson County, TN\"\t47089\n\"Sevier County, TN\"\t47155\t\"Knox County, TN\"\t47093\n\"Sevier County, TN\"\t47155\t\"Sevier County, TN\"\t47155\n\"Shelby County, TN\"\t47157\t\"Crittenden County, AR\"\t05035\n\"Shelby County, TN\"\t47157\t\"Mississippi County, AR\"\t05093\n\"Shelby County, TN\"\t47157\t\"DeSoto County, MS\"\t28033\n\"Shelby County, TN\"\t47157\t\"Marshall County, MS\"\t28093\n\"Shelby County, TN\"\t47157\t\"Fayette County, TN\"\t47047\n\"Shelby County, TN\"\t47157\t\"Shelby County, TN\"\t47157\n\"Shelby County, TN\"\t47157\t\"Tipton County, TN\"\t47167\n\"Smith County, TN\"\t47159\t\"DeKalb County, TN\"\t47041\n\"Smith County, TN\"\t47159\t\"Jackson County, TN\"\t47087\n\"Smith County, TN\"\t47159\t\"Macon County, TN\"\t47111\n\"Smith County, TN\"\t47159\t\"Putnam County, TN\"\t47141\n\"Smith County, TN\"\t47159\t\"Smith County, TN\"\t47159\n\"Smith County, TN\"\t47159\t\"Trousdale County, TN\"\t47169\n\"Smith County, TN\"\t47159\t\"Wilson County, TN\"\t47189\n\"Stewart County, TN\"\t47161\t\"Calloway County, KY\"\t21035\n\"Stewart County, TN\"\t47161\t\"Christian County, KY\"\t21047\n\"Stewart County, TN\"\t47161\t\"Trigg County, KY\"\t21221\n\"Stewart County, TN\"\t47161\t\"Benton County, TN\"\t47005\n\"Stewart County, TN\"\t47161\t\"Henry County, TN\"\t47079\n\"Stewart County, TN\"\t47161\t\"Houston County, TN\"\t47083\n\"Stewart County, TN\"\t47161\t\"Montgomery County, TN\"\t47125\n\"Stewart County, TN\"\t47161\t\"Stewart County, TN\"\t47161\n\"Sullivan County, TN\"\t47163\t\"Carter County, TN\"\t47019\n\"Sullivan County, TN\"\t47163\t\"Hawkins County, TN\"\t47073\n\"Sullivan County, TN\"\t47163\t\"Johnson County, TN\"\t47091\n\"Sullivan County, TN\"\t47163\t\"Sullivan County, TN\"\t47163\n\"Sullivan County, TN\"\t47163\t\"Washington County, TN\"\t47179\n\"Sullivan County, TN\"\t47163\t\"Scott County, VA\"\t51169\n\"Sullivan County, TN\"\t47163\t\"Washington County, VA\"\t51191\n\"Sullivan County, TN\"\t47163\t\"Bristol city, VA\"\t51520\n\"Sumner County, TN\"\t47165\t\"Allen County, KY\"\t21003\n\"Sumner County, TN\"\t47165\t\"Simpson County, KY\"\t21213\n\"Sumner County, TN\"\t47165\t\"Davidson County, TN\"\t47037\n\"Sumner County, TN\"\t47165\t\"Macon County, TN\"\t47111\n\"Sumner County, TN\"\t47165\t\"Robertson County, TN\"\t47147\n\"Sumner County, TN\"\t47165\t\"Sumner County, TN\"\t47165\n\"Sumner County, TN\"\t47165\t\"Trousdale County, TN\"\t47169\n\"Sumner County, TN\"\t47165\t\"Wilson County, TN\"\t47189\n\"Tipton County, TN\"\t47167\t\"Crittenden County, AR\"\t05035\n\"Tipton County, TN\"\t47167\t\"Mississippi County, AR\"\t05093\n\"Tipton County, TN\"\t47167\t\"Fayette County, TN\"\t47047\n\"Tipton County, TN\"\t47167\t\"Haywood County, TN\"\t47075\n\"Tipton County, TN\"\t47167\t\"Lauderdale County, TN\"\t47097\n\"Tipton County, TN\"\t47167\t\"Shelby County, TN\"\t47157\n\"Tipton County, TN\"\t47167\t\"Tipton County, TN\"\t47167\n\"Trousdale County, TN\"\t47169\t\"Macon County, TN\"\t47111\n\"Trousdale County, TN\"\t47169\t\"Smith County, TN\"\t47159\n\"Trousdale County, TN\"\t47169\t\"Sumner County, TN\"\t47165\n\"Trousdale County, TN\"\t47169\t\"Trousdale County, TN\"\t47169\n\"Trousdale County, TN\"\t47169\t\"Wilson County, TN\"\t47189\n\"Unicoi County, TN\"\t47171\t\"Madison County, NC\"\t37115\n\"Unicoi County, TN\"\t47171\t\"Mitchell County, NC\"\t37121\n\"Unicoi County, TN\"\t47171\t\"Yancey County, NC\"\t37199\n\"Unicoi County, TN\"\t47171\t\"Carter County, TN\"\t47019\n\"Unicoi County, TN\"\t47171\t\"Greene County, TN\"\t47059\n\"Unicoi County, TN\"\t47171\t\"Unicoi County, TN\"\t47171\n\"Unicoi County, TN\"\t47171\t\"Washington County, TN\"\t47179\n\"Union County, TN\"\t47173\t\"Anderson County, TN\"\t47001\n\"Union County, TN\"\t47173\t\"Campbell County, TN\"\t47013\n\"Union County, TN\"\t47173\t\"Claiborne County, TN\"\t47025\n\"Union County, TN\"\t47173\t\"Grainger County, TN\"\t47057\n\"Union County, TN\"\t47173\t\"Knox County, TN\"\t47093\n\"Union County, TN\"\t47173\t\"Union County, TN\"\t47173\n\"Van Buren County, TN\"\t47175\t\"Bledsoe County, TN\"\t47007\n\"Van Buren County, TN\"\t47175\t\"Cumberland County, TN\"\t47035\n\"Van Buren County, TN\"\t47175\t\"Sequatchie County, TN\"\t47153\n\"Van Buren County, TN\"\t47175\t\"Van Buren County, TN\"\t47175\n\"Van Buren County, TN\"\t47175\t\"Warren County, TN\"\t47177\n\"Van Buren County, TN\"\t47175\t\"White County, TN\"\t47185\n\"Warren County, TN\"\t47177\t\"Cannon County, TN\"\t47015\n\"Warren County, TN\"\t47177\t\"Coffee County, TN\"\t47031\n\"Warren County, TN\"\t47177\t\"DeKalb County, 
